vi "ConvertLabviewParameterToMatlabParamData.vi"(8 "BaseName":string, 9 "IgnoreContainerName":bool, 11 "Value":variant) -> (3 "Matlab Param Data":T1[](array[typedef]))   [LabVIEW 2017]
uses:
  LVPort/Matlab/Code/Methods/LVPortMatlabNamepathDataBundle.ctl
  LVPort/Matlab/VI/Methods/LVPortMatlabDataTypeEnum.ctl
  LVPort/Matlab/VI/Methods/LVPortMatlabContainerTypeEnum.ctl
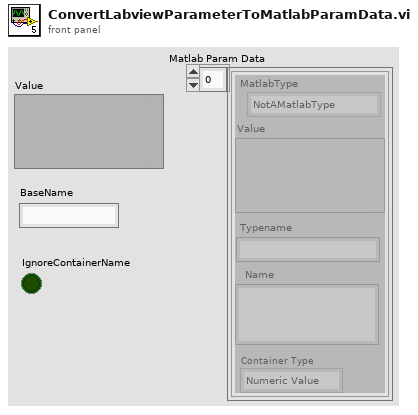
[diagram p1: front panel]
types:
  T1 = typedef "LVPortMatlabNamepathDataBundle.ctl" = cluster{"MatlabType":T2, "Value":variant, "Name":string, "Typename":string, "Container Type":T3}
  T2 = typedef "LVPortMatlabDataTypeEnum.ctl" = enum16{"NotAMatlabType", "Real", "Complex", "String", "Boolean"}
  T3 = typedef "LVPortMatlabContainerTypeEnum.ctl" = enum16{"Numeric Value", "Numeric Array", "Waveform"}
  T4 = typedef "NI_Data Type.lvlib/Data Type.ctl" = enum8{"Invalid Type", "Void", "I8", "I16", "I32", "I64", "U8", "U16", "U32", "U64", "Single Float", "Double Float", "Extended Float", "Single Complex", "Double Complex", "Extended Complex", "Enum U8", "Enum U16", "Enum U32", "Enum U64", "Single Float With Unit", "Double Float With Unit", "Extended Float With Unit", "Single Complex with Unit", "Double Complex with Unit", "Extended Complex with Unit", "Boolean", "String", "Path", "Picture", "Tag", "Array", "Cluster", "Variant", "LV Variant", "Waveform", "Timestamp", "Digital Waveform", "Digital Data", "ExpressData", "Refnum", "External Data", "VI", "Poly VI", "LabVIEW Class Instance", "Fixed Point"}
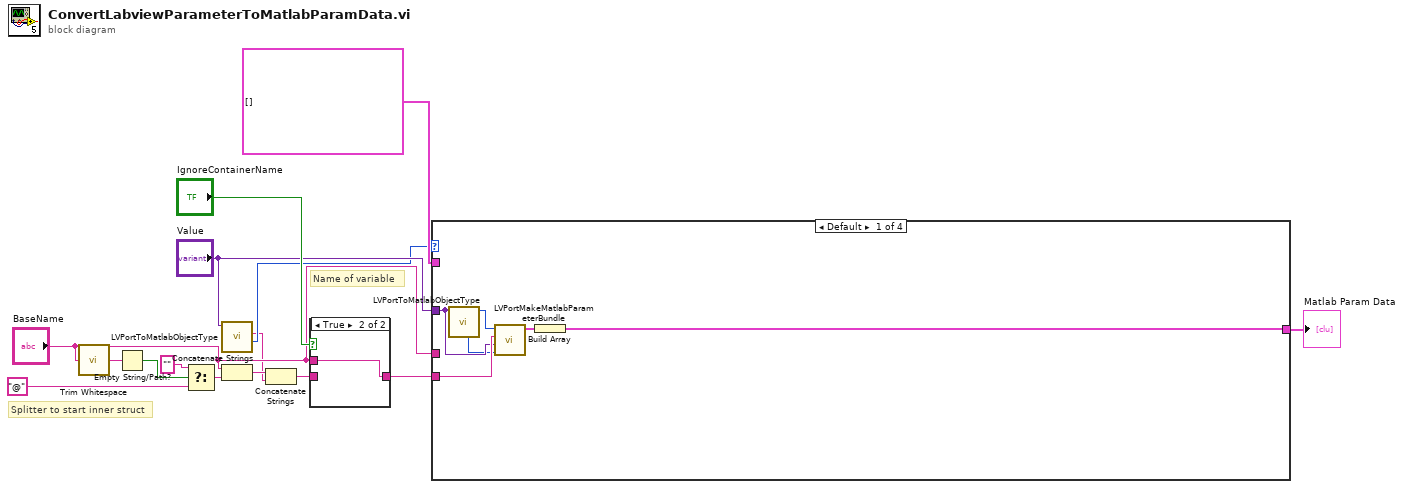
[diagram p0: block diagram]
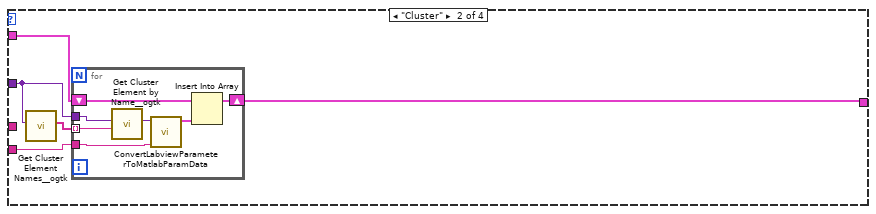
[diagram p3: hidden frame]
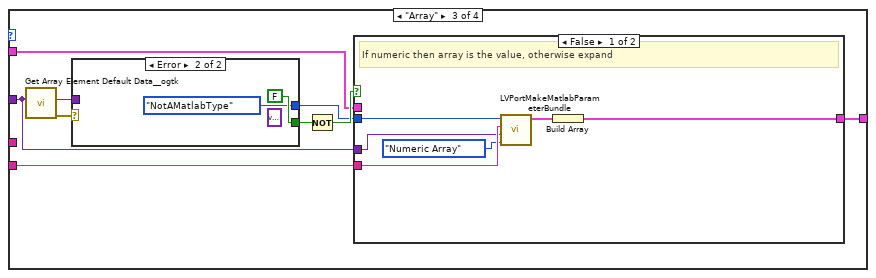
[diagram p4: hidden frame]
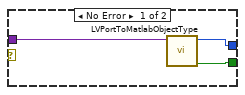
[diagram p5: hidden frame]
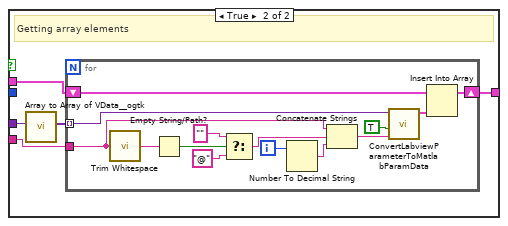
[diagram p6: hidden frame]
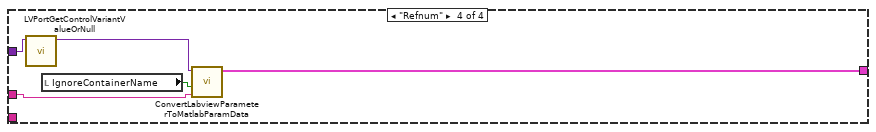
[diagram p7: hidden frame]
diagram:
  # "Splitter to start inner struct"
  # "Name of variable"
  n1 = call <vilib>:"Trim Whitespace.vi"("string"="BaseName") -> ("trimmed string"=w8:string)  [unwired: 1 in]
  n2 = Empty String/Path?(string/path=w8) -> (empty?=w7:bool)
  n3 = Select(t="" ("name"), s=w7, f="@" ("name")) -> (s? t:f=w15:string)
  n4 = call "LVPortToMatlabObjectType.vi"("Value"="Value") -> ("Type"=w2:T4, "Name"=w1:string)  [unwired: 6 in, 3 out]
  n5 = Concatenate Strings("BaseName", w15) -> (w9:string)
  n6 = Concatenate Strings(w9, w1) -> (w11:string)
  n7 = case shown="True" "IgnoreContainerName" {
    tunnel: [w16 w17] -> w12
    tunnel: w11 -> [w16 _]
    tunnel: "BaseName" -> [_ w17]
    frame False {
    }
    frame True {
    }
  }
  n8 = case shown="Default" w2 {
    tunnel: [w22 w28 w44 w77] -> w5
    tunnel: w12 -> [w20 w27 w41 _]
    tunnel: "BaseName" -> [_ _ _ w78]
    tunnel: T1[] [] -> [_ w25 w40 _]
    tunnel: "Value" -> [w19 w24 w39 w76]
    frame Default {
      n9 = call "LVPortToMatlabObjectType.vi"("Value"=w19) -> ("MatlabType"=w21:T2, "Container Type (Labview Value type)"=w18:T3)  [unwired: 6 in, 3 out]
      n10 = call "LVPortMakeMatlabParameterBundle.vi"("Labview Contriner type"=w18, "value"=w19, "name"=w20, "MatlabType"=w21) -> ("MatlabDataBundle"=w23:T1)  [unwired: 7 in]
      n11 = Build Array(w23) -> (w22:T1[])
    }
    frame "Cluster" {
      n12 = call <userlib>:"Get Cluster Element Names__ogtk.vi"("Cluster"=w24) -> ("Element Names"=w26:string[])  [unwired: 9 in, 1 out]
      n13 = for {
        shift-right: [w35] -> w28
        shift-left: w25 -> [w31]
        tunnel: w27 -> [w34]
        tunnel: w26 -> [w33] mode=indexing
        tunnel: w24 -> [w29]
        n14 = call <userlib>:"Get Cluster Element by Name__ogtk.vi"("Element Name"=w33, "Cluster"=w29) -> ("VElement"=w32:variant)  [unwired: 7 in, 2 out]
        n15 = call "ConvertLabviewParameterToMatlabParamData.vi"("BaseName"=w34, "Value"=w32) -> ("Matlab Param Data"=w30:T1[])  [unwired: 9 in]
        n16 = Insert Into Array(array=w31, new element=w30) -> (w35:T1[])  [unwired: 1 in]
      }
    }
    frame "Array" {
      n17 = call <userlib>:"Get Array Element Default Data__ogtk.vi"("Array"=w39) -> ("error out"=w38:errorcluster, "Array Element Default Data"=w36:variant)  [unwired: 9 in]
      n18 = case shown="Error" w38 {
        tunnel: [w47 FALSE ("IsNumeric")] -> w43
        tunnel: [w46 LVPortMatlabDataTypeEnum."NotAMatlabType" ("MatlabType")] -> w37
        tunnel: w36 -> [w45 _]
        frame No Error {
          n19 = call "LVPortToMatlabObjectType.vi"("Value"=w45) -> ("IsNumeric"=w47:bool, "MatlabType"=w46:T2)  [unwired: 6 in, 3 out]
        }
        frame Error {
          (unwired) variant
        }
      }
      n20 = Not(x=w43) -> (.not. x?=w42:bool)
      n21 = case shown="False" w42 {
        tunnel: [w53 w60] -> w44
        tunnel: w41 -> [w55 w59]
        tunnel: w40 -> [_ w58]
        tunnel: w39 -> [w52 w57]
        tunnel: w37 -> [w51 _]
        frame False {
          # "If numeric then array is the value, otherwise expand"
          n22 = call "LVPortMakeMatlabParameterBundle.vi"("Labview Contriner type"=LVPortMatlabContainerTypeEnum."Numeric Array", "value"=w52, "name"=w55, "MatlabType"=w51) -> ("MatlabDataBundle"=w54:T1)  [unwired: 7 in]
          n23 = Build Array(w54) -> (w53:T1[])
        }
        frame True {
          # "Getting array elements"
          n24 = call <userlib>:"Array to Array of VData__ogtk.vi"("MultiD Array"=w57) -> ("1D Array of Variants"=w56:variant[])  [unwired: 9 in, 1 out]
          n25 = for {
            shift-right: [w74] -> w60
            shift-left: w58 -> [w70]
            tunnel: w59 -> [w65]
            tunnel: w56 -> [w67] mode=indexing
            i -> [w68]
            n26 = call <vilib>:"Trim Whitespace.vi"("string"=w65) -> ("trimmed string"=w66:string)  [unwired: 1 in]
            n27 = Empty String/Path?(string/path=w66) -> (empty?=w64:bool)
            n28 = Select(t="", s=w64, f="@" ("string")) -> (s? t:f=w61:string)
            n29 = Number To Decimal String(number=w68) -> (decimal integer string=w73:string)  [unwired: 1 in]
            n30 = Concatenate Strings(w65, w61, w73) -> (w72:string)
            n31 = call "ConvertLabviewParameterToMatlabParamData.vi"("BaseName"=w72, "IgnoreContainerName"=TRUE, "Value"=w67) -> ("Matlab Param Data"=w69:T1[])  [unwired: 8 in]
            n32 = Insert Into Array(array=w70, new element=w69) -> (w74:T1[])  [unwired: 1 in]
          }
        }
      }
    }
    frame "Refnum" {
      n33 = call "LVPortGetControlVariantValueOrNull.vi"("ControlVariant"=w76) -> ("Value"=w79:variant)  [unwired: 9 in, 1 out]
      n34 = local read "IgnoreContainerName"() -> (w75:bool)
      n35 = call "ConvertLabviewParameterToMatlabParamData.vi"("BaseName"=w78, "IgnoreContainerName"=w75, "Value"=w79) -> ("Matlab Param Data"=w77:T1[])  [unwired: 8 in]
    }
  }
  "Matlab Param Data" <- w5
